vi "Do.vi"(8 "error in (no error)":errorcluster, 10 "Actor In":refnum<class "Actor.lvclass">, 11 "Enqueue Data Msg in":refnum<class "Enqueue Data Msg.lvclass">) -> (0 "error out":errorcluster, 1 "Stop Actor":bool, 2 "Actor Out":refnum<class "Actor.lvclass">)   [LabVIEW 2020, in "Scratchpad.lvlib" / "Test 1.lvlib" / "Enqueue Data Msg.lvclass"]
uses:
  Enqueue Data Msg.lvclass
  962aee91-99e7-462d-9c90-130c0ae2d8a7.vi
  Test 1/Test 1.lvclass
  Artifex/Actor/Actor.lvclass
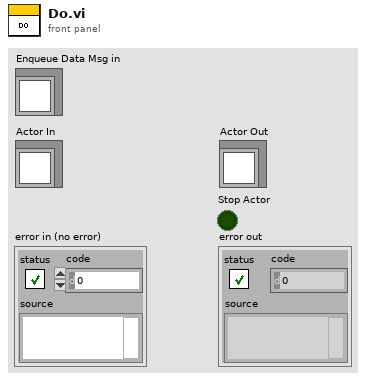
[diagram p1: front panel]
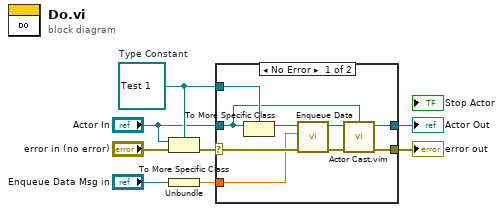
[diagram p0: block diagram]
diagram:
  w6 = refnum<class "Test 1.lvclass"> refnum  # Type Constant
  n1 = To More Specific Class(target class=w6, reference="Actor In", error in="error in (no error)") -> (error out=w7:errorcluster)  [unwired: 1 out]
  n2 = Unbundle("Enqueue Data Msg in") -> (w8:dbl)
  n3 = case shown="No Error" w7 {
    selector: w7 -> [w17 w18]
    tunnel: [w13 w19] -> w1
    tunnel: [w10 w18] -> w2
    tunnel: w8 -> [w15 _]
    tunnel: w6 -> [w11 _]
    tunnel: "Actor In" -> [w9 w19]
    frame No Error {
      n4 = To More Specific Class(target class=w11, reference=w9) -> (specific class reference=w14:refnum<class "Test 1.lvclass">)  [unwired: 1 in, 1 out]
      n5 = call "Enqueue Data.vi"("error in (no error)"=w17, "Data"=w15, "Test 1 in"=w14) -> ("error out"=w12:errorcluster, "Test 1 out"=w16:refnum<class "Test 1.lvclass">)  [unwired: 7 in]
      n6 = call "Actor Cast.vim"("Type"=w9, "Actor in"=w16, "error in (no error)"=w12) -> ("Actor out"=w13:refnum<class "Actor.lvclass">, "error out"=w10:errorcluster)  [unwired: 6 in]
    }
    frame Error {
    }
  }
  "error out" <- w2
  "Actor Out" <- w1
